vi "Stream Data.vi"(8 "error in (no error)":errorcluster, 9 "notifier out":refnum<notifier>, 10 "queue out":refnum<queue>, 11 "DAQ_msgHandler StreamTypeDef":T1) -> (0 "error out":errorcluster, 2 "Timout Counter":i32, 3 "DAQ_msgHandler StreamTypeDef 2":T1)   [LabVIEW 2024, in "DAQ_msgHandler Logging.lvlib"]
doc: "This VI uses the TDMS Write function to write data to a TDMS file."
uses:
  Logging/DAQ_msgHandler Logging.lvlib
  controls/DAQ_msgHandler StreamTypeDef.ctl
  CTRsample/Control/streamIO_states.ctl
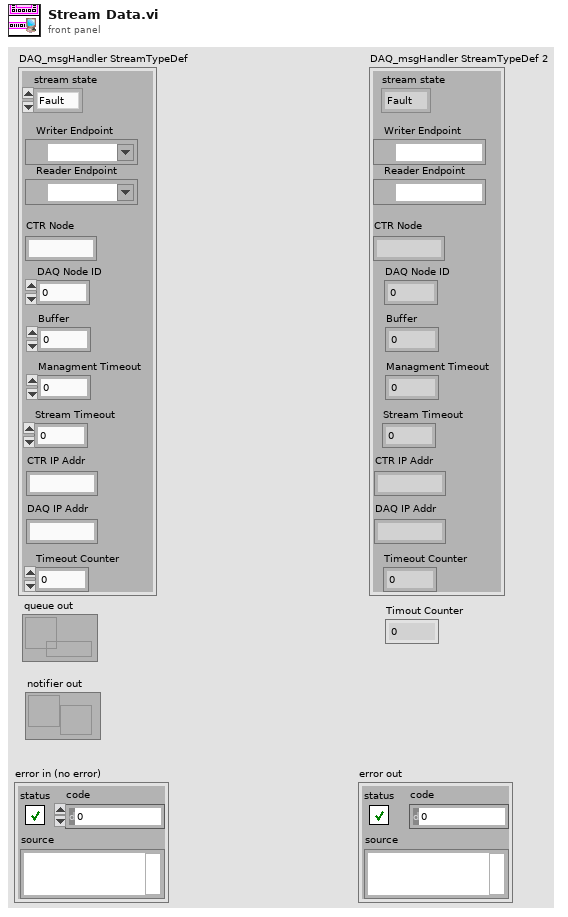
[diagram p1: front panel]
types:
  T1 = typedef "DAQ_msgHandler StreamTypeDef.ctl" = cluster{"stream state":T2, "CTR Node":string, "DAQ Node ID":i32, "Writer Endpoint":refnum<k21>, "Reader Endpoint":refnum<k21>, "Buffer":i32, "Managment Timeout":i32, "Stream Timeout":i32, "DAQ IP Addr":string, "CTR IP Addr":string, "Timeout Counter":i32}
  T2 = typedef "streamIO_states.ctl" = enum16{"Fault", "Initialize", "Stream", "Close"}
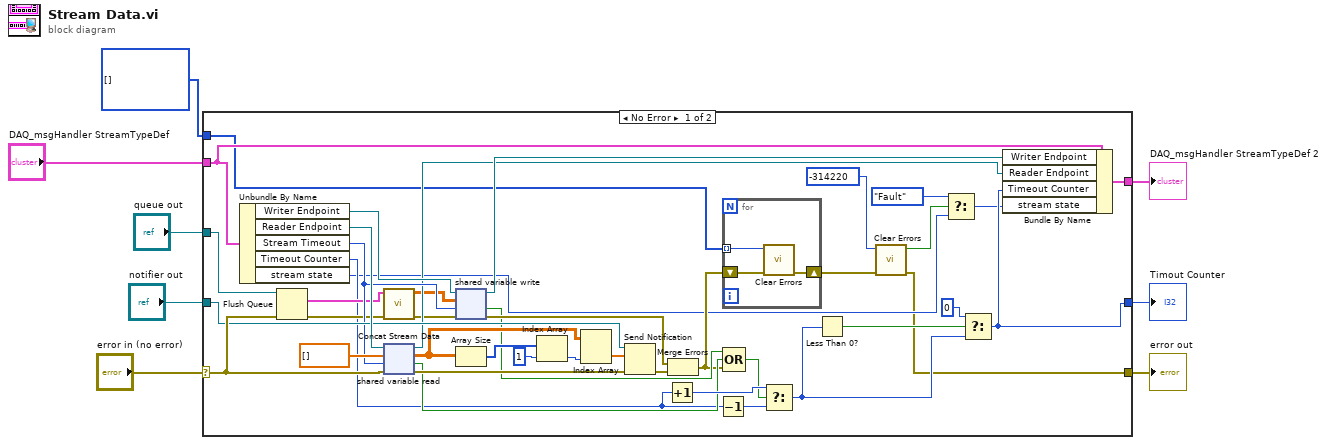
[diagram p0: block diagram]
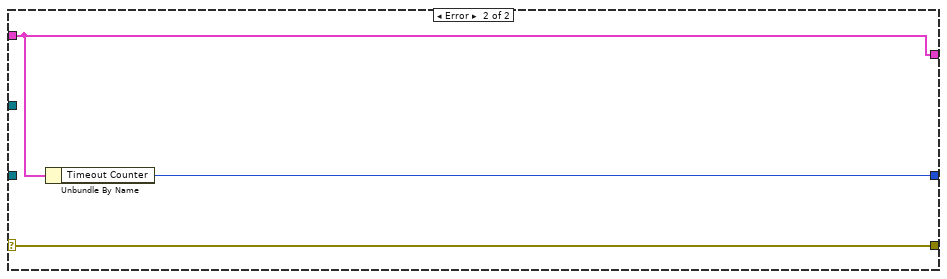
[diagram p2: hidden frame]
diagram:
  n1 = case shown="No Error" "error in (no error)" {
    selector: "error in (no error)" -> [w47 w56]
    tunnel: "queue out" -> [w48 _]
    tunnel: [w9 w56] -> w8
    tunnel: "DAQ_msgHandler StreamTypeDef" -> [w37 w55]
    tunnel: "notifier out" -> [w39 _]
    tunnel: [w36 w55] -> w5
    tunnel: i32[] [] -> [w18 _]
    tunnel: [w16 w54] -> w1
    frame No Error {
      n2 = Unbundle By Name(w37) -> ("Writer Endpoint"=w49:refnum<k21>, "Reader Endpoint"=w46:refnum<k21>, "Stream Timeout"=w38:i32, "Timeout Counter"=w19:i32, "stream state"=w10:T2)
      n3 = Flush Queue(queue=w48, error in (no error)=w47) -> (remaining elements=w30:cluster{"Stream/Aquire Data":dbl[][]}[], error out=w32:errorcluster)  [unwired: 1 out]
      n4 = call "Concat Stream Data.vi"("error in (no error)"=w32, "remaining elements"=w30) -> ("error out"=w31:errorcluster, "Stream/Aquire Data"=w29:dbl[][])  [unwired: 8 in]
      n5 = shared-variable-read(w46, w47, dbl[] [], w38) -> (w34:refnum<k21>, w44:errorcluster, w24:bool, w41:dbl[][])  [unwired: 1 in]
      n6 = shared-variable-write(w49, w31, w29, w38) -> (w35:refnum<k21>, w50:errorcluster, w25:bool)
      n7 = Array Size(array=w41) -> (size(s)=w42:i32[])
      n8 = Index Array(array=w42, index=1) -> (element=w40:i32)
      n9 = Index Array(array=w41, index (col)=w40) -> (element=w33:dbl[])  [unwired: 1 in]
      n10 = Send Notification(notification=w33, notifier=w39, error in (no error)=w44) -> (error out=w43:errorcluster)  [unwired: 1 out]
      n11 = Increment(x=w19) -> (x+1=w27:i32)
      n12 = Merge Errors(w50, w43) -> (w17:errorcluster)
      n13 = Decrement(x=w19) -> (x-1=w23:i32)
      n14 = for {
        shift-right: [w52] -> w15
        shift-left: w17 -> [w53]
        tunnel: w18 -> [w51] mode=indexing
        n15 = call <vilib>:"Clear Errors.vi"("error in (no error)"=w53, "specific error code to clear (0: all)"=w51) -> ("error out"=w52:errorcluster)  [unwired: 4 in, 1 out]
      }
      n16 = Compound Arithmetic op=OR(w25, w24, w17) -> (w26:bool)
      n17 = Select(t=w27, s=w26, f=w23) -> (s? t:f=w20:i32)
      n18 = Less Than 0?(x=w20) -> (x < 0?=w22:bool)
      n19 = call <vilib>:"Clear Errors.vi"("error in (no error)"=w15, "specific error code to clear (0: all)"=-314220) -> ("error out"=w9:errorcluster, "specific error cleared?"=w13:bool)  [unwired: 4 in]
      n20 = Select(t=streamIO_states."Fault" ("stream state"), s=w13, f=w10) -> (s? t:f=w11:T2)
      n21 = Select(t=0 ("f"), s=w22, f=w20) -> (s? t:f=w16:i32)
      n22 = Bundle By Name(cluster=w37, "Writer Endpoint"=w35, "Reader Endpoint"=w34, "Timeout Counter"=w16, "stream state"=w11) -> (w36:T1)
    }
    frame Error {
      n23 = Unbundle By Name(w55) -> ("Timeout Counter"=w54:i32)
    }
  }
  "error out" <- w8
  "DAQ_msgHandler StreamTypeDef 2" <- w5
  "Timout Counter" <- w1
